vi "Autonomous Independent.vi"   [LabVIEW 2019]
doc: "This VI is called when autonomous begins, and will automatically be terminated when autonomous ends. You can carry out timed or sensor driven robot movement independently without needing to return to the caller."
uses:
  <vilib>/addons/control/pid/NI_PID_pid.lvlib
  <vilib>/Rock Robotics/WPI/SafetyOutput/WPI_SafetyOutputConfigMenu.ctl
  <vilib>/Rock Robotics/Network Tables/NT Write Numeric Array.vi
  <vilib>/addons/control/pid/pid.llb/PID (DBL).vi
types:
  T1 = typedef "WPI_SafetyOutputConfigMenu.ctl" = enum16{"Enable", "Disable"}
  T2 = typedef "WPI_JoystickDevRef.ctl" = cluster{"Device":T3}
  T3 = typedef "WPI_JoystickDeviceEnum.ctl" = enum16{"USB 0", "USB 1", "USB 2", "USB 3", "USB 4", "USB 5"}
  T4 = typedef "WPI_MotorControlDeviceRef.ctl" = cluster{"DeviceStatus":errorcluster, "Type":T5, "PWM":cluster{"PWM Channel":T6, "DeadBand":T7}, "CAN":cluster{"Device Number":u8, "SetOutput VI Ref":variant, "GetOutput VI Ref":variant, "Enable VI Ref":variant, "Disable VI Ref":variant, "Data":variant}, "Invert":bool, "DIO PWM":cluster{"PWM \"Enable\" Channel":T6, "DIOChannel":T8, "PWM Rate":dbl}}
  T5 = typedef "WPI_MotorControlType.ctl" = enum16{"PWM", "CAN", "DIO PWM"}
  T6 = typedef "FPGA_DIOPWMChannel.ctl" = enum8{"PWM 0", "PWM 1", "PWM 2", "PWM 3", "PWM 4", "PWM 5", "PWM 6", "PWM 7", "PWM 8", "PWM 9", "PWM MXP 0", "PWM MXP 1", "PWM MXP 2", "PWM MXP 3", "PWM MXP 4", "PWM MXP 5", "PWM MXP 6", "PWM MXP 7", "PWM MXP 8", "PWM MXP 9", "Invalid"}
  T7 = typedef "WPI_PWMDeadband.ctl" = cluster{"Name":string, "maxPositivePwm":i32, "minPositivePwm":i32, "centerPwm":i32, "maxNegativePwm":i32, "minNegativePwm":i32, "angularRange":u16}
  T8 = typedef "FPGA_DIOChannel.ctl" = enum8{"DIO 0", "DIO 1", "DIO 2", "DIO 3", "DIO 4", "DIO 5", "DIO 6", "DIO 7", "DIO 8", "DIO 9", "DIO MXP 0", "DIO MXP 1", "DIO MXP 2", "DIO MXP 3", "DIO MXP 4", "DIO MXP 5", "DIO MXP 6", "DIO MXP 7", "DIO MXP 8", "DIO MXP 9", "DIO MXP 10", "DIO MXP 11", "DIO MXP 12", "DIO MXP 13", "DIO MXP 14", "DIO MXP 15", "SPI Port CS1", "SPI Port CS2", "SPI Port CS3", "SPI Port MISO", "SPI Port MOSI", "Invalid"}
  T9 = typedef "WPI_DigitalInputDevRef.ctl" = cluster{"DevStatus":errorcluster, "DIO Channel":T8}
  T10 = cluster{"proportional gain (Kc)":dbl, "integral time (Ti, min)":dbl, "derivative time (Td, min)":dbl}
  T11 = cluster{"Yaw":dbl, "Roll":dbl, "Pitch":dbl, "Heading":dbl, "Fused Heading":dbl}
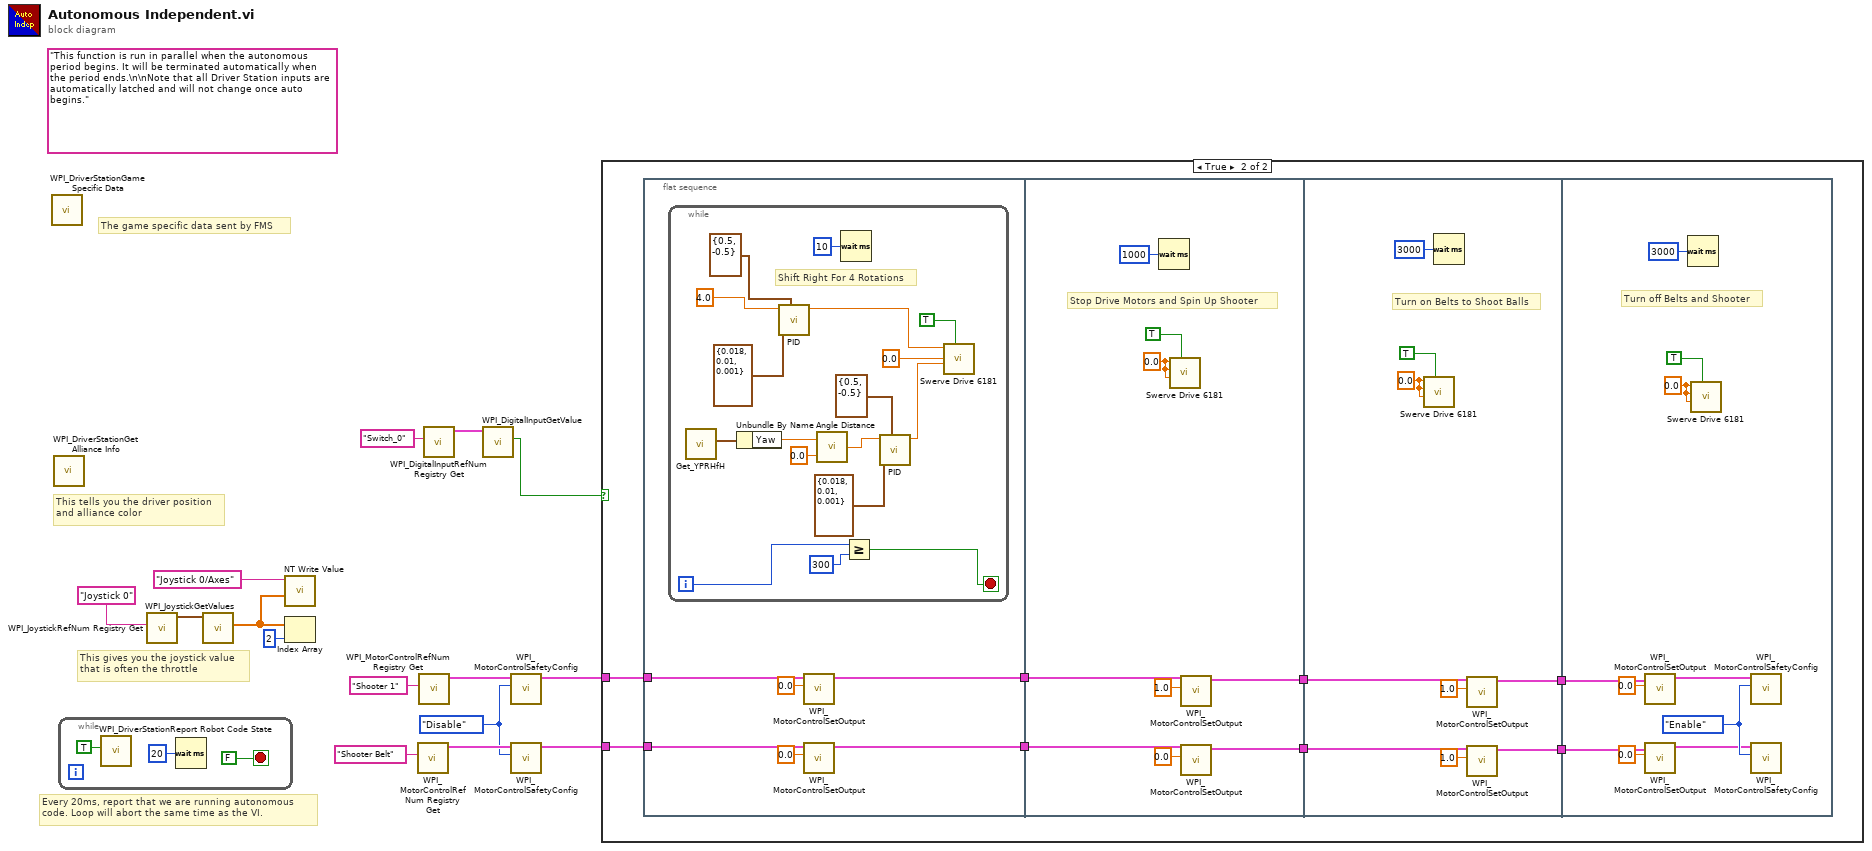
[diagram p0: block diagram]
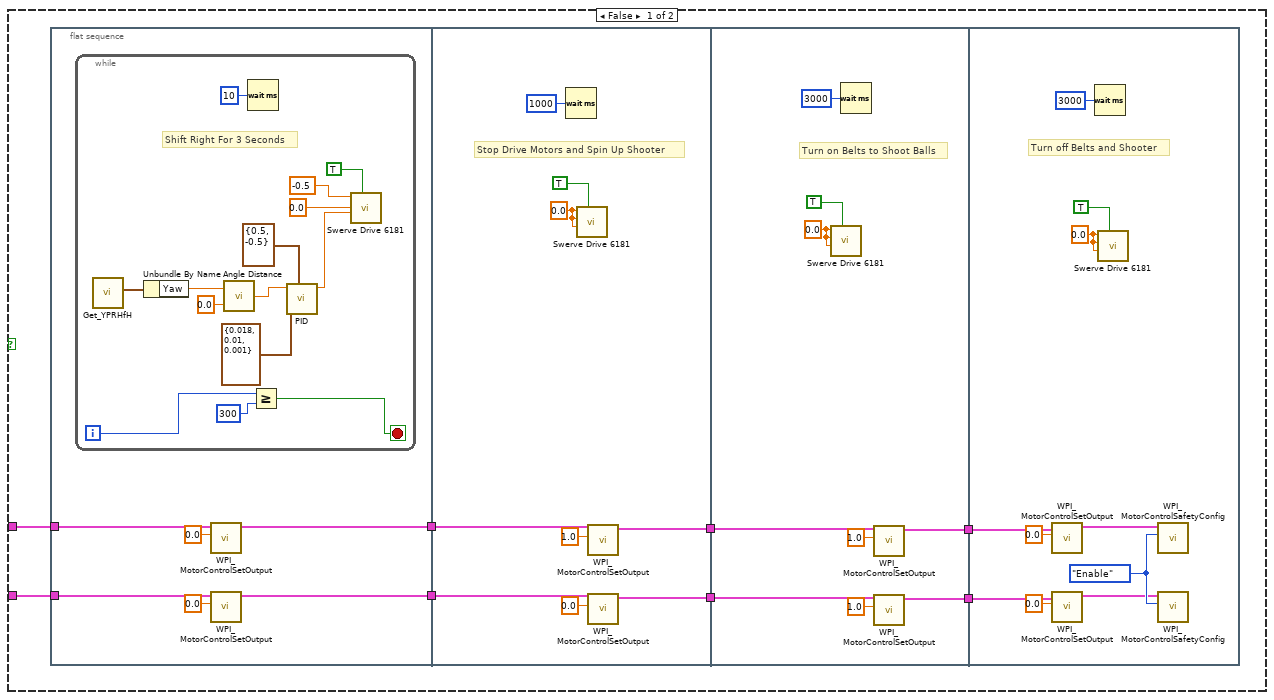
[diagram p2: hidden frame]
diagram:
  w6 = WPI_SafetyOutputConfigMenu."Disable" ("mode")
  (unwired) "This function is run in parallel when the autonomous period begins. It will be terminated automatically when the period ends.\n\nNote that all Driver Station inputs are automatically latched and will not change once auto begins."
  # "The game specific data sent by FMS"
  # "Every 20ms, report that we are running autonomous\ncode. Loop will abort the same time as the VI."
  # "This gives you the joystick value\nthat is often the throttle"
  # "This tells you the driver position\nand alliance color"
  n1 = call <vilib>:"WPI_DriverStationGame Specific Data.vi"() -> ()  [unwired: 11 in, 1 out]
  n2 = call <vilib>:"WPI_DriverStationGet Alliance Info.vi"() -> ()  [unwired: 12 out]
  n3 = while {
    stop <- FALSE stop-if-true
    n4 = call <vilib>:"WPI_DriverStationReport Robot Code State.vi"("Autonomous"=TRUE) -> ()  [unwired: 10 in, 1 out]
    n5 = Wait (ms)(milliseconds to wait=u32 20) -> ()  [unwired: 1 out]
  }
  n6 = call <vilib>:"WPI_JoystickRefNum Registry Get.vi"("refnum name"="Joystick 0") -> ("JoystickDevRef"=w14:T2)  [unwired: 1 in, 9 out]
  n7 = call <vilib>:"WPI_JoystickGetValues.vi"("JoystickDevRef"=w14) -> ("Axes"=w12:dbl[])  [unwired: 6 in, 4 out]
  n8 = call-poly <vilib>:"NT Write Value.vi"("Numeric Array"=w12, "Name"="Joystick 0/Axes") -> ()  [unwired: 9 in, 1 out]
  n9 = Index Array(array=w12, index=2) -> ()  [unwired: 1 out]
  n10 = call <vilib>:"WPI_MotorControlRefNum Registry Get.vi"("refnum name"="Shooter Belt") -> ("MotorControlDevRef"=w8:T4)  [unwired: 9 in, 1 out]
  n11 = call <vilib>:"WPI_MotorControlRefNum Registry Get.vi"("refnum name"="Shooter 1") -> ("MotorControlDevRef"=w7:T4)  [unwired: 9 in, 1 out]
  n12 = call <vilib>:"WPI_DigitalInputRefNum Registry Get.vi"("refnum name"="Switch_0") -> ("DigitalInputDevRef"=w3:T9)  [unwired: 9 in, 1 out]
  n13 = call <vilib>:"WPI_DigitalInputGetValue.vi"("DigitalInputDevRef"=w3) -> ("Value"=w2:bool)  [unwired: 8 in, 2 out]
  n14 = call <vilib>:"WPI_MotorControlSafetyConfig.vi"("mode"=w6, "MotorControlDevRef"=w7) -> ("MotorControlDevRef"=w4:T4)  [unwired: 8 in, 1 out]
  n15 = call <vilib>:"WPI_MotorControlSafetyConfig.vi"("mode"=w6, "MotorControlDevRef"=w8) -> ("MotorControlDevRef"=w5:T4)  [unwired: 8 in, 1 out]
  n16 = case shown="True" w2 {
    tunnel: w5 -> [w20 w76]
    tunnel: w4 -> [w19 w75]
    frame False {
      n17 = flat-sequence {
        tunnel: w20 -> [w32]
        tunnel: w19 -> [w31]
        tunnel: [w28] -> w26
        tunnel: [w27] -> w25
        tunnel: w26 -> [w52]
        tunnel: w25 -> [w51]
        tunnel: [w50] -> w24
        tunnel: [w49] -> w23
        tunnel: w24 -> [w63]
        tunnel: w23 -> [w62]
        tunnel: [w61] -> w22
        tunnel: [w60] -> w21
        tunnel: w22 -> [w73]
        tunnel: w21 -> [w72]
        frame #0 {
          n18 = while {
            i -> [w45]
            stop <- w44 stop-if-true
            # "Shift Right For 3 Seconds"
            n19 = call <vilib>:"Get_YPRHfH.vi"() -> ("YRPHfH"=w41:T11)  [unwired: 11 in]
            n20 = Unbundle By Name(w41) -> ("Yaw"=w40:dbl)
            n21 = call "Angle Distance.vi"("target angle"=0.0, "current angle"=w40) -> ("distance"=w42:dbl)
            n22 = Wait (ms)(milliseconds to wait=u32 10) -> ()  [unwired: 1 out]
            n23 = Greater Or Equal?(x=w45, y=300) -> (x >= y?=w44:bool)
            n24 = call-poly <vilib>:"PID.vi"("output range"=cluster{"output high":dbl, "output low":dbl} {"output high"=0.5, "output low"=-0.5}, "PID gains"=T10 {"proportional gain (Kc)"=0.018, "integral time (Ti, min)"=0.01, "derivative time (Td, min)"=0.001}, "setpoint"=w42) -> ("output"=w38:dbl)  [unwired: 7 in, 1 out]
            n25 = call "Swerve Drive 6181.vi"("X"=-0.5, "Y"=0.0, "Z"=w38, "Auto Controls"=TRUE) -> ()  [unwired: 3 in]
          }
          n26 = call <vilib>:"WPI_MotorControlSetOutput.vi"("Output"=0.0, "MotorControlDevRef"=w31) -> ("MotorControlDevRef"=w28:T4)  [unwired: 7 in, 2 out]
          n27 = call <vilib>:"WPI_MotorControlSetOutput.vi"("Output"=0.0, "MotorControlDevRef"=w32) -> ("MotorControlDevRef"=w27:T4)  [unwired: 7 in, 2 out]
        }
        frame #1 {
          w54 = 0.0 ("X")
          # "Stop Drive Motors and Spin Up Shooter"
          n28 = Wait (ms)(milliseconds to wait=u32 1000) -> ()  [unwired: 1 out]
          n29 = call "Swerve Drive 6181.vi"("X"=w54, "Y"=w54, "Z"=w54, "Auto Controls"=TRUE) -> ()  [unwired: 3 in]
          n30 = call <vilib>:"WPI_MotorControlSetOutput.vi"("Output"=1.0, "MotorControlDevRef"=w52) -> ("MotorControlDevRef"=w50:T4)  [unwired: 7 in, 2 out]
          n31 = call <vilib>:"WPI_MotorControlSetOutput.vi"("Output"=0.0, "MotorControlDevRef"=w51) -> ("MotorControlDevRef"=w49:T4)  [unwired: 7 in, 2 out]
        }
        frame #2 {
          w57 = 0.0 ("X")
          # "Turn on Belts to Shoot Balls"
          n32 = call "Swerve Drive 6181.vi"("X"=w57, "Y"=w57, "Z"=w57, "Auto Controls"=TRUE) -> ()  [unwired: 3 in]
          n33 = Wait (ms)(milliseconds to wait=u32 3000) -> ()  [unwired: 1 out]
          n34 = call <vilib>:"WPI_MotorControlSetOutput.vi"("Output"=1.0, "MotorControlDevRef"=w63) -> ("MotorControlDevRef"=w61:T4)  [unwired: 7 in, 2 out]
          n35 = call <vilib>:"WPI_MotorControlSetOutput.vi"("Output"=1.0, "MotorControlDevRef"=w62) -> ("MotorControlDevRef"=w60:T4)  [unwired: 7 in, 2 out]
        }
        frame #3 {
          w65 = 0.0 ("X")
          w69 = WPI_SafetyOutputConfigMenu."Enable" ("mode")
          # "Turn off Belts and Shooter"
          n36 = call <vilib>:"WPI_MotorControlSetOutput.vi"("Output"=0.0, "MotorControlDevRef"=w73) -> ("MotorControlDevRef"=w68:T4)  [unwired: 7 in, 2 out]
          n37 = call <vilib>:"WPI_MotorControlSetOutput.vi"("Output"=0.0, "MotorControlDevRef"=w72) -> ("MotorControlDevRef"=w67:T4)  [unwired: 7 in, 2 out]
          n38 = Wait (ms)(milliseconds to wait=u32 3000) -> ()  [unwired: 1 out]
          n39 = call "Swerve Drive 6181.vi"("X"=w65, "Y"=w65, "Z"=w65, "Auto Controls"=TRUE) -> ()  [unwired: 3 in]
          n40 = call <vilib>:"WPI_MotorControlSafetyConfig.vi"("mode"=w69, "MotorControlDevRef"=w68) -> ()  [unwired: 8 in, 2 out]
          n41 = call <vilib>:"WPI_MotorControlSafetyConfig.vi"("mode"=w69, "MotorControlDevRef"=w67) -> ()  [unwired: 8 in, 2 out]
        }
      }
    }
    frame True {
      n42 = flat-sequence {
        tunnel: w76 -> [w88]
        tunnel: w75 -> [w87]
        tunnel: [w84] -> w82
        tunnel: [w83] -> w81
        tunnel: w82 -> [w111]
        tunnel: w81 -> [w110]
        tunnel: [w109] -> w80
        tunnel: [w108] -> w79
        tunnel: w80 -> [w122]
        tunnel: w79 -> [w121]
        tunnel: [w120] -> w78
        tunnel: [w119] -> w77
        tunnel: w78 -> [w132]
        tunnel: w77 -> [w131]
        frame #0 {
          n43 = while {
            i -> [w104]
            stop <- w103 stop-if-true
            # "Shift Right For 4 Rotations"
            n44 = call <vilib>:"Get_YPRHfH.vi"() -> ("YRPHfH"=w100:T11)  [unwired: 11 in]
            n45 = Unbundle By Name(w100) -> ("Yaw"=w99:dbl)
            n46 = call-poly <vilib>:"PID.vi"("output range"=cluster{"output high":dbl, "output low":dbl} {"output high"=0.5, "output low"=-0.5}, "PID gains"=T10 {"proportional gain (Kc)"=0.018, "integral time (Ti, min)"=0.01, "derivative time (Td, min)"=0.001}, "setpoint"=4.0) -> ("output"=w90:dbl)  [unwired: 7 in, 1 out]
            n47 = call "Angle Distance.vi"("target angle"=0.0, "current angle"=w99) -> ("distance"=w101:dbl)
            n48 = Wait (ms)(milliseconds to wait=u32 10) -> ()  [unwired: 1 out]
            n49 = Greater Or Equal?(x=w104, y=300) -> (x >= y?=w103:bool)
            n50 = call-poly <vilib>:"PID.vi"("output range"=cluster{"output high":dbl, "output low":dbl} {"output high"=0.5, "output low"=-0.5}, "PID gains"=T10 {"proportional gain (Kc)"=0.018, "integral time (Ti, min)"=0.01, "derivative time (Td, min)"=0.001}, "setpoint"=w101) -> ("output"=w97:dbl)  [unwired: 7 in, 1 out]
            n51 = call "Swerve Drive 6181.vi"("X"=w90, "Y"=0.0, "Z"=w97, "Auto Controls"=TRUE) -> ()  [unwired: 3 in]
          }
          n52 = call <vilib>:"WPI_MotorControlSetOutput.vi"("Output"=0.0, "MotorControlDevRef"=w87) -> ("MotorControlDevRef"=w84:T4)  [unwired: 7 in, 2 out]
          n53 = call <vilib>:"WPI_MotorControlSetOutput.vi"("Output"=0.0, "MotorControlDevRef"=w88) -> ("MotorControlDevRef"=w83:T4)  [unwired: 7 in, 2 out]
        }
        frame #1 {
          w113 = 0.0 ("X")
          # "Stop Drive Motors and Spin Up Shooter"
          n54 = Wait (ms)(milliseconds to wait=u32 1000) -> ()  [unwired: 1 out]
          n55 = call "Swerve Drive 6181.vi"("X"=w113, "Y"=w113, "Z"=w113, "Auto Controls"=TRUE) -> ()  [unwired: 3 in]
          n56 = call <vilib>:"WPI_MotorControlSetOutput.vi"("Output"=1.0, "MotorControlDevRef"=w111) -> ("MotorControlDevRef"=w109:T4)  [unwired: 7 in, 2 out]
          n57 = call <vilib>:"WPI_MotorControlSetOutput.vi"("Output"=0.0, "MotorControlDevRef"=w110) -> ("MotorControlDevRef"=w108:T4)  [unwired: 7 in, 2 out]
        }
        frame #2 {
          w116 = 0.0 ("X")
          # "Turn on Belts to Shoot Balls"
          n58 = call "Swerve Drive 6181.vi"("X"=w116, "Y"=w116, "Z"=w116, "Auto Controls"=TRUE) -> ()  [unwired: 3 in]
          n59 = Wait (ms)(milliseconds to wait=u32 3000) -> ()  [unwired: 1 out]
          n60 = call <vilib>:"WPI_MotorControlSetOutput.vi"("Output"=1.0, "MotorControlDevRef"=w122) -> ("MotorControlDevRef"=w120:T4)  [unwired: 7 in, 2 out]
          n61 = call <vilib>:"WPI_MotorControlSetOutput.vi"("Output"=1.0, "MotorControlDevRef"=w121) -> ("MotorControlDevRef"=w119:T4)  [unwired: 7 in, 2 out]
        }
        frame #3 {
          w124 = 0.0 ("X")
          w128 = WPI_SafetyOutputConfigMenu."Enable" ("mode")
          # "Turn off Belts and Shooter"
          n62 = call <vilib>:"WPI_MotorControlSetOutput.vi"("Output"=0.0, "MotorControlDevRef"=w132) -> ("MotorControlDevRef"=w127:T4)  [unwired: 7 in, 2 out]
          n63 = call <vilib>:"WPI_MotorControlSetOutput.vi"("Output"=0.0, "MotorControlDevRef"=w131) -> ("MotorControlDevRef"=w126:T4)  [unwired: 7 in, 2 out]
          n64 = Wait (ms)(milliseconds to wait=u32 3000) -> ()  [unwired: 1 out]
          n65 = call "Swerve Drive 6181.vi"("X"=w124, "Y"=w124, "Z"=w124, "Auto Controls"=TRUE) -> ()  [unwired: 3 in]
          n66 = call <vilib>:"WPI_MotorControlSafetyConfig.vi"("mode"=w128, "MotorControlDevRef"=w127) -> ()  [unwired: 8 in, 2 out]
          n67 = call <vilib>:"WPI_MotorControlSafetyConfig.vi"("mode"=w128, "MotorControlDevRef"=w126) -> ()  [unwired: 8 in, 2 out]
        }
      }
    }
  }
